vi "Profile Auton - Distance.vi"(8 "error in (no error)":errorcluster, 10 "Time (s)":dbl format="%#_13g", 11 "Distance (ft)":dbl) -> (0 "error out":errorcluster)   [LabVIEW 2017]
uses:
  Robot Global Data.vi
  <vilib>/Rock Robotics/Network Tables/NT Write Number.vi
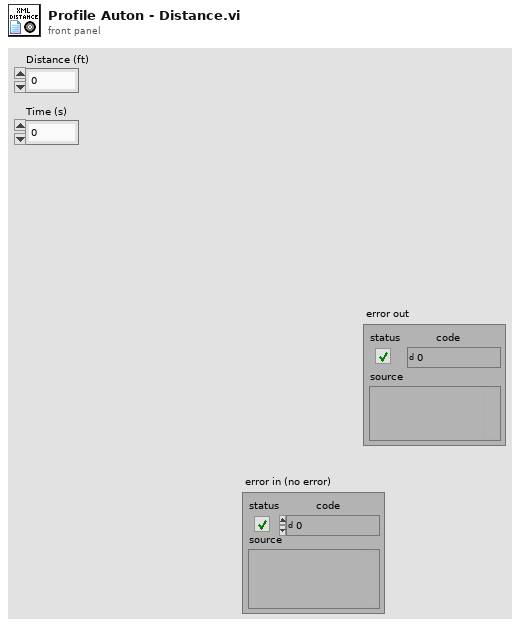
[diagram p1: front panel]
types:
  T1 = typedef "WPI_MotorControlDeviceRef.ctl" = cluster{"DeviceStatus":errorcluster, "Type":T2, "PWM":cluster{"PWM Channel":T3, "DeadBand":T4}, "CAN":cluster{"Device Number":u8, "SetOutput VI Ref":variant, "GetOutput VI Ref":variant, "Enable VI Ref":variant, "Disable VI Ref":variant, "Data":variant}, "Invert":bool, "DIO PWM":cluster{"PWM \"Enable\" Channel":T3, "DIOChannel":T5, "PWM Rate":dbl}}
  T2 = typedef "WPI_MotorControlType.ctl" = enum16{"PWM", "CAN", "DIO PWM"}
  T3 = typedef "FPGA_DIOPWMChannel.ctl" = enum8{"PWM 0", "PWM 1", "PWM 2", "PWM 3", "PWM 4", "PWM 5", "PWM 6", "PWM 7", "PWM 8", "PWM 9", "PWM MXP 0", "PWM MXP 1", "PWM MXP 2", "PWM MXP 3", "PWM MXP 4", "PWM MXP 5", "PWM MXP 6", "PWM MXP 7", "PWM MXP 8", "PWM MXP 9", "Invalid"}
  T4 = typedef "WPI_PWMDeadband.ctl" = cluster{"Name":string, "maxPositivePwm":i32, "minPositivePwm":i32, "centerPwm":i32, "maxNegativePwm":i32, "minNegativePwm":i32, "angularRange":u16}
  T5 = typedef "FPGA_DIOChannel.ctl" = enum8{"DIO 0", "DIO 1", "DIO 2", "DIO 3", "DIO 4", "DIO 5", "DIO 6", "DIO 7", "DIO 8", "DIO 9", "DIO MXP 0", "DIO MXP 1", "DIO MXP 2", "DIO MXP 3", "DIO MXP 4", "DIO MXP 5", "DIO MXP 6", "DIO MXP 7", "DIO MXP 8", "DIO MXP 9", "DIO MXP 10", "DIO MXP 11", "DIO MXP 12", "DIO MXP 13", "DIO MXP 14", "DIO MXP 15", "SPI Port CS1", "SPI Port CS2", "SPI Port CS3", "SPI Port MISO", "SPI Port MOSI", "Invalid"}
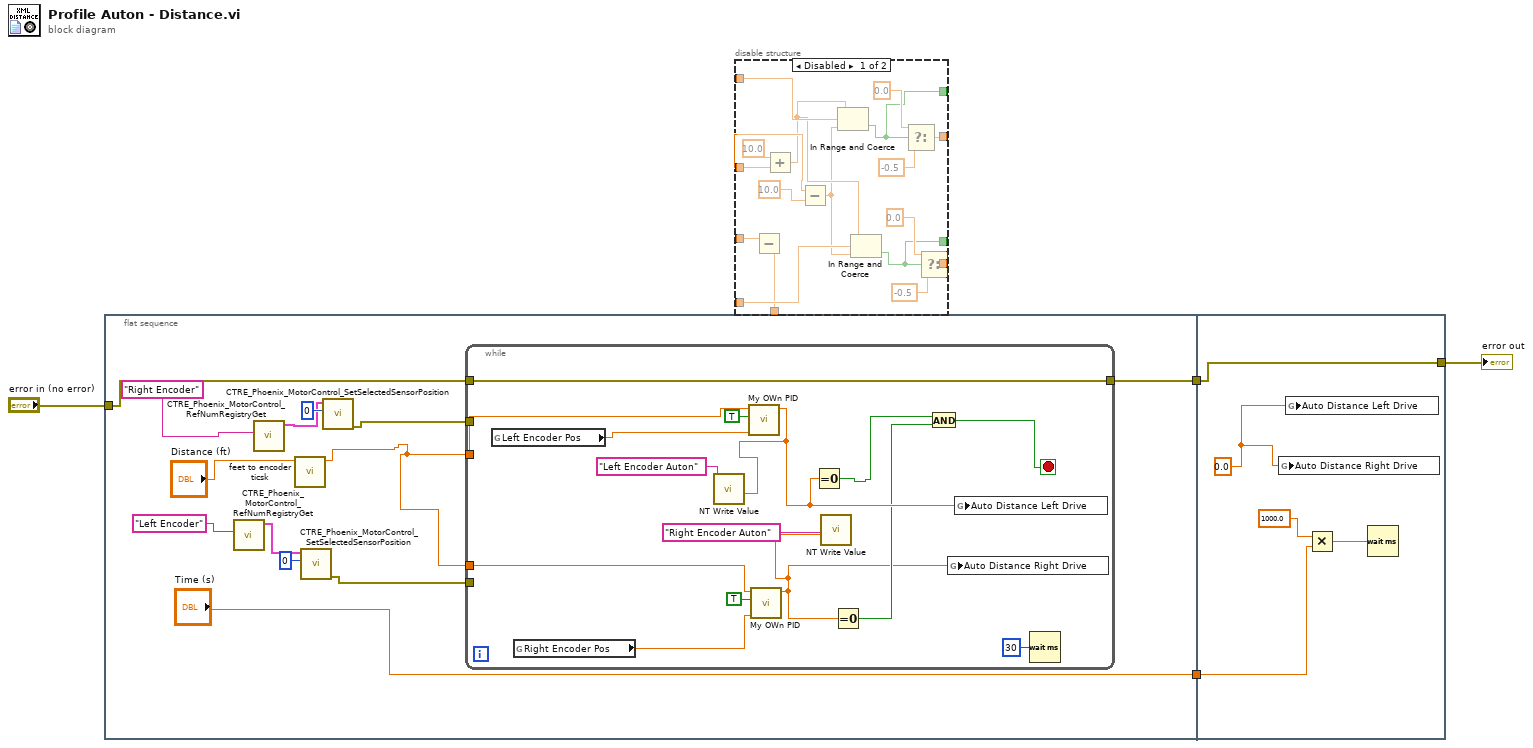
[diagram p0: block diagram]
diagram:
  n1 = flat-sequence {
    tunnel: ["Time (s)"] -> w4
    tunnel: "error in (no error)" -> [w15]
    tunnel: [w14] -> w2
    tunnel: w4 -> [w36]
    tunnel: w2 -> [w33]
    tunnel: [w33] -> w1
    frame #0 {
      n2 = call <vilib>:"CTRE_Phoenix_MotorControl_RefNumRegistryGet.vi"("refnum name"="Left Encoder") -> ("PhoenixMotorControlDevRef"=w6:T1)  [unwired: 9 in, 1 out]
      n3 = call <vilib>:"CTRE_Phoenix_MotorControl_RefNumRegistryGet.vi"("refnum name"="Right Encoder") -> ("PhoenixMotorControlDevRef"=w7:T1)  [unwired: 9 in, 1 out]
      n4 = call "feet to encoder ticsk.vi"("Distance in feet wanted"="Distance (ft)") -> ("Encoder Ticks"=w13:dbl)  [unwired: 10 in]
      n5 = call <vilib>:"CTRE_Phoenix_MotorControl_SetSelectedSensorPosition.vi"("New Sensor Position"=0, "PhoenixMotorControlDevRef"=w6) -> ("error out"=w12:errorcluster)  [unwired: 8 in, 1 out]
      n6 = call <vilib>:"CTRE_Phoenix_MotorControl_SetSelectedSensorPosition.vi"("New Sensor Position"=0, "PhoenixMotorControlDevRef"=w7) -> ("error out"=w9:errorcluster)  [unwired: 8 in, 1 out]
      n7 = while {
        tunnel: w13 -> [w30]
        tunnel: w13 -> [w29]
        tunnel: w15 -> [w28]
        tunnel: [w28] -> w14
        tunnel: w12 -> [_]
        tunnel: w9 -> [_]
        stop <- w32 stop-if-true
        n8 = global read "Robot Global Data.vi" "Left Encoder Pos"() -> (w25:dbl)
        n9 = global read "Robot Global Data.vi" "Right Encoder Pos"() -> (w24:dbl)
        n10 = call "My OWn PID.vi"("Current Input"=w25, "Encoders (t) gyro (f)"=TRUE, "Wanted End"=w29) -> ("Output"=w20:dbl)  [unwired: 8 in]
        n11 = call-poly <vilib>:"NT Write Value.vi"("Numeric"=w20, "Name"="Left Encoder Auton") -> ()  [unwired: 9 in, 1 out]
        n12 = call "My OWn PID.vi"("Current Input"=w24, "Encoders (t) gyro (f)"=TRUE, "Wanted End"=w30) -> ("Output"=w18:dbl)  [unwired: 8 in]
        n13 = Equal To 0?(x=w20) -> (x = 0?=w21:bool)
        n14 = call-poly <vilib>:"NT Write Value.vi"("Numeric"=w18, "Name"="Right Encoder Auton") -> ()  [unwired: 9 in, 1 out]
        n15 = Equal To 0?(x=w18) -> (x = 0?=w19:bool)
        n16 = And(x=w21, y=w19) -> (x .and. y?=w32:bool)
        n17 = global write "Robot Global Data.vi" "Auto Distance Right Drive"(w18) -> ()
        n18 = global write "Robot Global Data.vi" "Auto Distance Left Drive"(w20) -> ()
        n19 = Wait (ms)(milliseconds to wait=u32 30) -> ()  [unwired: 1 out]
      }
    }
    frame #1 {
      w34 = 0.0
      n20 = global write "Robot Global Data.vi" "Auto Distance Right Drive"(w34) -> ()
      n21 = global write "Robot Global Data.vi" "Auto Distance Left Drive"(w34) -> ()
      n22 = Multiply(x=1000.0, y=w36) -> (x*y=w37:dbl)
      n23 = Wait (ms)(milliseconds to wait=w37) -> ()  [unwired: 1 out]
    }
  }
  n24 = disable-structure shown="Disabled" {
    disable-tunnel: _ -> [w52 _]
    disable-tunnel: _ -> [w50 _]
    disable-tunnel: _ -> [w46 _]
    disable-tunnel: [w43 _] -> _
    disable-tunnel: [w42 _] -> _
    disable-tunnel: [w41 _] -> _
    disable-tunnel: [w40 _] -> _
    disable-tunnel: _ -> [w39 _]
    disable-tunnel: [w38 _] -> _
    frame Disabled {
      n25 = Subtract(x=w39) -> (x-y=w38:dbl)  [unwired: 1 in]
      n26 = Add(x=10.0, y=w50) -> (x+y=w45:dbl)
      n27 = Subtract(x=w50, y=10.0) -> (x-y=w44:dbl)
      n28 = In Range and Coerce(upper limit=w45, x=w52, lower limit=w44) -> (In Range?=w43:bool)  [unwired: 1 out]
      n29 = In Range and Coerce(upper limit=w45, x=w46, lower limit=w44) -> (In Range?=w42:bool)  [unwired: 1 out]
      n30 = Select(t=0.0, s=w43, f=-0.5) -> (s? t:f=w41:dbl)
      n31 = Select(t=0.0, s=w42, f=-0.5) -> (s? t:f=w40:dbl)
    }
    frame Enabled {
    }
  }
  "error out" <- w1
